vi "stepped_inflation.vi"() -> ()   [LabVIEW 2014]
doc: "This VI demonstrates the individual configuration of settings in I/W, W/I, and continuous operation modes.\n\nThis VI is not meant to be used with infusion-only models. \n\nNotes:\n(1) If continuous mode is selected, infuse volumes/rates will be used."
uses:
  <instrlib>/KD Scientific 2XX Series/KD Scientific 2XX Series.lvlib
panel:
  in  "number of steps":i32
  out "Units":string
  out "Delivered Volume":dbl
  in  "stop":bool
  out "Status":T1
  in  "Baud Rate (9600)":u32(ring)=9600 items=["300"=300, "1200"=1200, "2400"=2400, "4800"=4800, "9600"=9600]
  in  "Withdrawal Settings":T2={"Flow Rate (5)"=5.0, "Volume (10)"=10.0, "Volume Units (ml)"=enum."milliliters (ml)", "Rate Units (ml/min.)"=enum."milliliters per minute (ml/min.)"} {"Volume (10)" format="%#.3g"}
  in  "Diameter (8.75 mm)":dbl=8.75
  in  "Infusion Settings":T2={"Flow Rate (5)"=5.0, "Volume (10)"=10.0, "Volume Units (ml)"=enum."milliliters (ml)", "Rate Units (ml/min.)"=enum."milliliters per minute (ml/min.)"}
  in  "Operation Mode (Infuse)":u16(ring) items=["Infuse", "Withdraw", "Infuse-Withdraw", "Withdraw-Infuse", "Continuous"]
  in  "Address (0)":i32 format="%0.0f"
  in  "error in (no error)":errorcluster
  in  "VISA resource name":refnum<visa-resource-name>="COM1"
  # "© 2005 National Instruments Corporation.  ALL RIGHTS RESERVED."
  # "RS-232 Settings"
  # "General Settings"
  # "Pump Status"
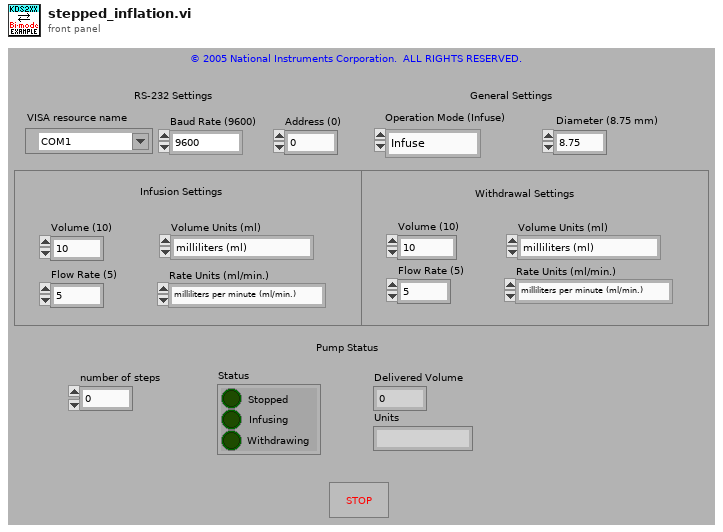
[diagram p1: front panel]
types:
  T1 = cluster{"Stopped":bool, "Infusing":bool, "Withdrawing":bool}
  T2 = cluster{"Flow Rate (5)":dbl, "Volume (10)":dbl, "Volume Units (ml)":enum16{"milliliters (ml)", "microliters (ul)"}, "Rate Units (ml/min.)":enum16{"milliliters per minute (ml/min.)", "milliliters per hour (ml/hr.)", "microliters per minute (ul/min.)", "microliters per hour (ul/hr.)"}}
  T3 = enum16{"milliliters per minute (ml/min.)", "milliliters per hour (ml/hr.)", "microliters per minute (ul/min.)", "microliters per hour (ul/hr.)"}
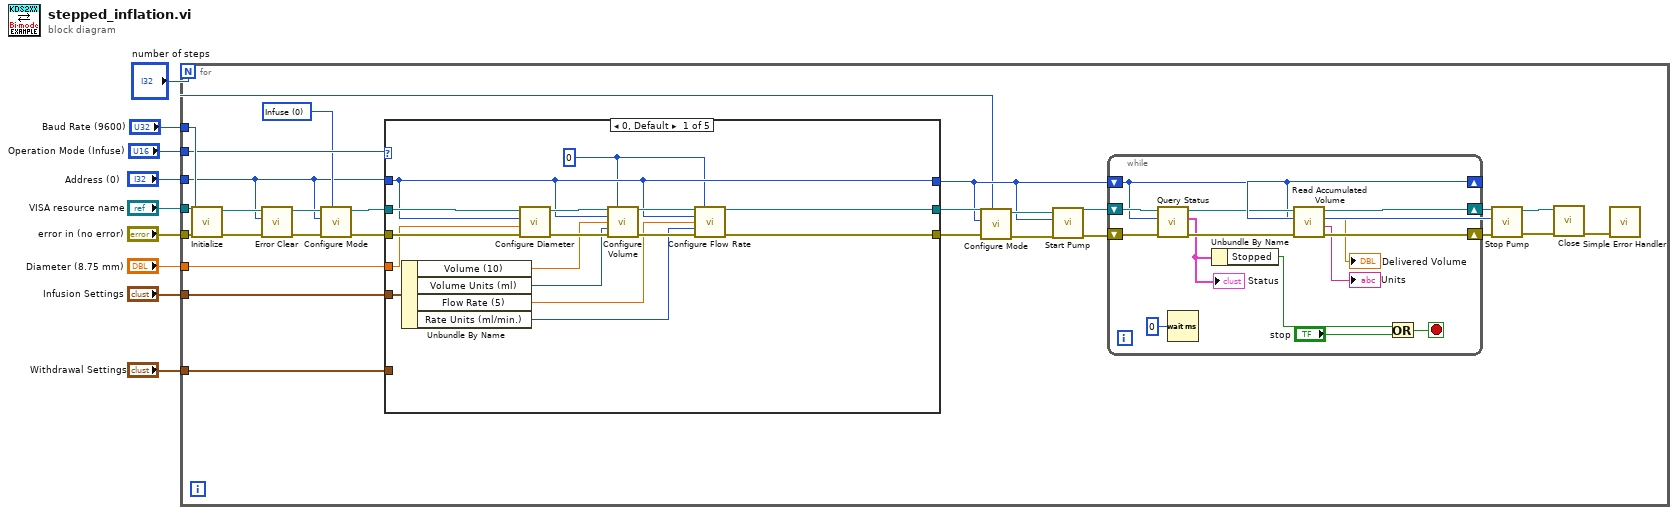
[diagram p0: block diagram]
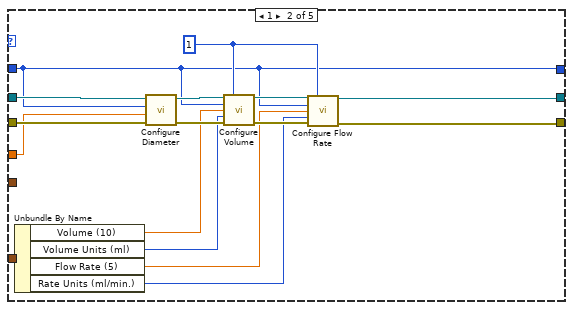
[diagram p2: hidden frame]
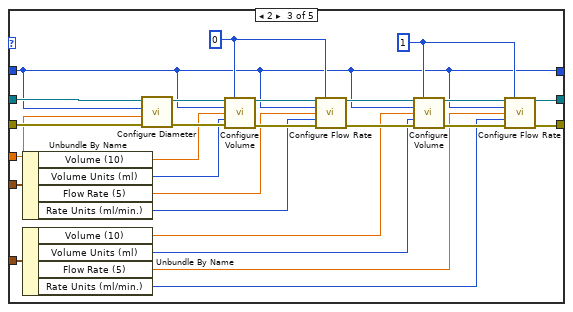
[diagram p3: hidden frame]
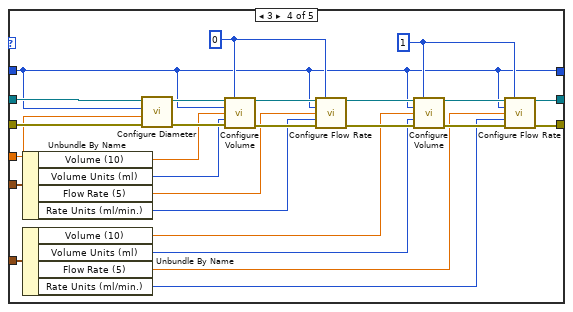
[diagram p4: hidden frame]
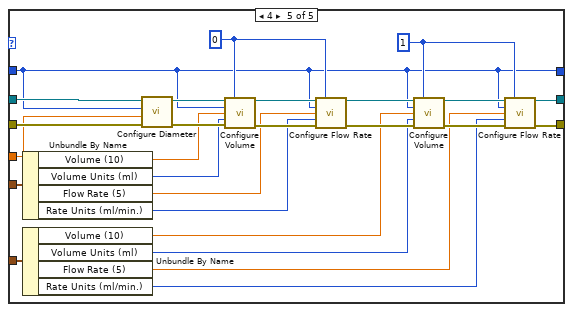
[diagram p5: hidden frame]
diagram:
  n1 = for {
    N: "number of steps" -> [_]
    tunnel: "VISA resource name" -> [w37]
    tunnel: "error in (no error)" -> [w36]
    tunnel: "Infusion Settings" -> [w31]
    tunnel: "Withdrawal Settings" -> [w30]
    tunnel: "Diameter (8.75 mm)" -> [w29]
    tunnel: "Baud Rate (9600)" -> [w24]
    tunnel: "Operation Mode (Infuse)" -> [w18]
    tunnel: "Address (0)" -> [w10]
    w15 = u16 0 items=["Infuse", "Withdraw", "Infuse-Withdraw", "Withdraw-Infuse", "Continuous"] ("Mode (infuse)")
    n2 = call <instrlib>:"Initialize.vi"("error in (no error)"=w36, "Baud Rate (9600)"=w24, "VISA resource name"=w37) -> ("error out"=w12:errorcluster, "VISA resource name out"=w11:refnum<visa-resource-name>)  [unwired: 7 in]
    n3 = call <instrlib>:"Error Clear.vi"("error in (no error)"=w12, "Address (0)"=w10, "VISA resource name"=w11) -> ("error out"=w13:errorcluster, "VISA resource name out"=w14:refnum<visa-resource-name>)  [unwired: 6 in, 1 out]
    n4 = call <instrlib>:"Configure Mode.vi"("Mode (infuse)"=w15, "error in (no error)"=w13, "Address (0)"=w10, "VISA resource name"=w14) -> ("error out"=w17:errorcluster, "VISA resource name out"=w16:refnum<visa-resource-name>)  [unwired: 6 in]
    n5 = case shown="0, Default" w18 {
      tunnel: w31 -> [w47 _ w95 w121 w147]
      tunnel: w30 -> [_ w69 w94 w120 w146]
      tunnel: w16 -> [w53 w68 w93 w119 w145]
      tunnel: w17 -> [w52 w64 w92 w118 w144]
      tunnel: w29 -> [w46 w60 w75 w101 w127]
      tunnel: [w45 w54 w70 w96 w122] -> w19
      tunnel: w10 -> [w45 w54 w70 w96 w122]
      tunnel: [w40 w65 w72 w98 w124] -> w23
      tunnel: [w39 w61 w71 w97 w123] -> w22
      frame 0, Default {
        w38 = 0
        n6 = Unbundle By Name(w47) -> ("Volume (10)"=w44:dbl, "Volume Units (ml)"=w43:enum16{"milliliters (ml)", "microliters (ul)"}, "Flow Rate (5)"=w42:dbl, "Rate Units (ml/min.)"=w41:T3)
        n7 = call <instrlib>:"Configure Diameter.vi"("error in (no error)"=w52, "Diameter (8.75 mm)"=w46, "Address (0)"=w45, "VISA resource name"=w53) -> ("error out"=w50:errorcluster, "VISA resource name out"=w51:refnum<visa-resource-name>)  [unwired: 6 in]
        n8 = call <instrlib>:"Configure Volume.vi"("VISA resource name"=w51, "Mode (infuse)"=w38, "Address (0)"=w45, "Volume (100)"=w44, "Units (0: milliliters)"=w43, "error in (no error)"=w50) -> ("VISA resource name out"=w49:refnum<visa-resource-name>, "error out"=w48:errorcluster)  [unwired: 8 in]
        n9 = call <instrlib>:"Configure Flow Rate.vi"("VISA resource name"=w49, "Mode (infuse)"=w38, "Address (0)"=w45, "Flow Rate (5)"=w42, "Units (0: milliliters per minute)"=w41, "error in (no error)"=w48) -> ("VISA resource name out"=w40:refnum<visa-resource-name>, "error out"=w39:errorcluster)  [unwired: 8 in]
      }
      frame 1 {
        w55 = 1
        n10 = Unbundle By Name(w69) -> ("Volume (10)"=w59:dbl, "Volume Units (ml)"=w58:enum16{"milliliters (ml)", "microliters (ul)"}, "Flow Rate (5)"=w57:dbl, "Rate Units (ml/min.)"=w56:T3)
        n11 = call <instrlib>:"Configure Diameter.vi"("error in (no error)"=w64, "Diameter (8.75 mm)"=w60, "Address (0)"=w54, "VISA resource name"=w68) -> ("error out"=w63:errorcluster, "VISA resource name out"=w67:refnum<visa-resource-name>)  [unwired: 6 in]
        n12 = call <instrlib>:"Configure Volume.vi"("VISA resource name"=w67, "Mode (infuse)"=w55, "Address (0)"=w54, "Volume (100)"=w59, "Units (0: milliliters)"=w58, "error in (no error)"=w63) -> ("VISA resource name out"=w66:refnum<visa-resource-name>, "error out"=w62:errorcluster)  [unwired: 8 in]
        n13 = call <instrlib>:"Configure Flow Rate.vi"("VISA resource name"=w66, "Mode (infuse)"=w55, "Address (0)"=w54, "Flow Rate (5)"=w57, "Units (0: milliliters per minute)"=w56, "error in (no error)"=w62) -> ("VISA resource name out"=w65:refnum<visa-resource-name>, "error out"=w61:errorcluster)  [unwired: 8 in]
      }
      frame 2 {
        w73 = 1
        w74 = 0
        n14 = Unbundle By Name(w95) -> ("Volume (10)"=w83:dbl, "Volume Units (ml)"=w82:enum16{"milliliters (ml)", "microliters (ul)"}, "Flow Rate (5)"=w81:dbl, "Rate Units (ml/min.)"=w80:T3)
        n15 = Unbundle By Name(w94) -> ("Volume (10)"=w79:dbl, "Volume Units (ml)"=w78:enum16{"milliliters (ml)", "microliters (ul)"}, "Flow Rate (5)"=w77:dbl, "Rate Units (ml/min.)"=w76:T3)
        n16 = call <instrlib>:"Configure Diameter.vi"("error in (no error)"=w92, "Diameter (8.75 mm)"=w75, "Address (0)"=w70, "VISA resource name"=w93) -> ("error out"=w87:errorcluster, "VISA resource name out"=w91:refnum<visa-resource-name>)  [unwired: 6 in]
        n17 = call <instrlib>:"Configure Volume.vi"("VISA resource name"=w91, "Mode (infuse)"=w74, "Address (0)"=w70, "Volume (100)"=w83, "Units (0: milliliters)"=w82, "error in (no error)"=w87) -> ("VISA resource name out"=w90:refnum<visa-resource-name>, "error out"=w86:errorcluster)  [unwired: 8 in]
        n18 = call <instrlib>:"Configure Flow Rate.vi"("VISA resource name"=w90, "Mode (infuse)"=w74, "Address (0)"=w70, "Flow Rate (5)"=w81, "Units (0: milliliters per minute)"=w80, "error in (no error)"=w86) -> ("VISA resource name out"=w89:refnum<visa-resource-name>, "error out"=w85:errorcluster)  [unwired: 8 in]
        n19 = call <instrlib>:"Configure Volume.vi"("VISA resource name"=w89, "Mode (infuse)"=w73, "Address (0)"=w70, "Volume (100)"=w79, "Units (0: milliliters)"=w78, "error in (no error)"=w85) -> ("VISA resource name out"=w88:refnum<visa-resource-name>, "error out"=w84:errorcluster)  [unwired: 8 in]
        n20 = call <instrlib>:"Configure Flow Rate.vi"("VISA resource name"=w88, "Mode (infuse)"=w73, "Address (0)"=w70, "Flow Rate (5)"=w77, "Units (0: milliliters per minute)"=w76, "error in (no error)"=w84) -> ("VISA resource name out"=w72:refnum<visa-resource-name>, "error out"=w71:errorcluster)  [unwired: 8 in]
      }
      frame 3 {
        w99 = 1
        w100 = 0
        n21 = Unbundle By Name(w121) -> ("Volume (10)"=w109:dbl, "Volume Units (ml)"=w108:enum16{"milliliters (ml)", "microliters (ul)"}, "Flow Rate (5)"=w107:dbl, "Rate Units (ml/min.)"=w106:T3)
        n22 = Unbundle By Name(w120) -> ("Volume (10)"=w105:dbl, "Volume Units (ml)"=w104:enum16{"milliliters (ml)", "microliters (ul)"}, "Flow Rate (5)"=w103:dbl, "Rate Units (ml/min.)"=w102:T3)
        n23 = call <instrlib>:"Configure Diameter.vi"("error in (no error)"=w118, "Diameter (8.75 mm)"=w101, "Address (0)"=w96, "VISA resource name"=w119) -> ("error out"=w113:errorcluster, "VISA resource name out"=w117:refnum<visa-resource-name>)  [unwired: 6 in]
        n24 = call <instrlib>:"Configure Volume.vi"("VISA resource name"=w117, "Mode (infuse)"=w100, "Address (0)"=w96, "Volume (100)"=w109, "Units (0: milliliters)"=w108, "error in (no error)"=w113) -> ("VISA resource name out"=w116:refnum<visa-resource-name>, "error out"=w112:errorcluster)  [unwired: 8 in]
        n25 = call <instrlib>:"Configure Flow Rate.vi"("VISA resource name"=w116, "Mode (infuse)"=w100, "Address (0)"=w96, "Flow Rate (5)"=w107, "Units (0: milliliters per minute)"=w106, "error in (no error)"=w112) -> ("VISA resource name out"=w115:refnum<visa-resource-name>, "error out"=w111:errorcluster)  [unwired: 8 in]
        n26 = call <instrlib>:"Configure Volume.vi"("VISA resource name"=w115, "Mode (infuse)"=w99, "Address (0)"=w96, "Volume (100)"=w105, "Units (0: milliliters)"=w104, "error in (no error)"=w111) -> ("VISA resource name out"=w114:refnum<visa-resource-name>, "error out"=w110:errorcluster)  [unwired: 8 in]
        n27 = call <instrlib>:"Configure Flow Rate.vi"("VISA resource name"=w114, "Mode (infuse)"=w99, "Address (0)"=w96, "Flow Rate (5)"=w103, "Units (0: milliliters per minute)"=w102, "error in (no error)"=w110) -> ("VISA resource name out"=w98:refnum<visa-resource-name>, "error out"=w97:errorcluster)  [unwired: 8 in]
      }
      frame 4 {
        w125 = 1
        w126 = 0
        n28 = Unbundle By Name(w147) -> ("Volume (10)"=w135:dbl, "Volume Units (ml)"=w134:enum16{"milliliters (ml)", "microliters (ul)"}, "Flow Rate (5)"=w133:dbl, "Rate Units (ml/min.)"=w132:T3)
        n29 = Unbundle By Name(w146) -> ("Volume (10)"=w131:dbl, "Volume Units (ml)"=w130:enum16{"milliliters (ml)", "microliters (ul)"}, "Flow Rate (5)"=w129:dbl, "Rate Units (ml/min.)"=w128:T3)
        n30 = call <instrlib>:"Configure Diameter.vi"("error in (no error)"=w144, "Diameter (8.75 mm)"=w127, "Address (0)"=w122, "VISA resource name"=w145) -> ("error out"=w139:errorcluster, "VISA resource name out"=w143:refnum<visa-resource-name>)  [unwired: 6 in]
        n31 = call <instrlib>:"Configure Volume.vi"("VISA resource name"=w143, "Mode (infuse)"=w126, "Address (0)"=w122, "Volume (100)"=w135, "Units (0: milliliters)"=w134, "error in (no error)"=w139) -> ("VISA resource name out"=w142:refnum<visa-resource-name>, "error out"=w138:errorcluster)  [unwired: 8 in]
        n32 = call <instrlib>:"Configure Flow Rate.vi"("VISA resource name"=w142, "Mode (infuse)"=w126, "Address (0)"=w122, "Flow Rate (5)"=w133, "Units (0: milliliters per minute)"=w132, "error in (no error)"=w138) -> ("VISA resource name out"=w141:refnum<visa-resource-name>, "error out"=w137:errorcluster)  [unwired: 8 in]
        n33 = call <instrlib>:"Configure Volume.vi"("VISA resource name"=w141, "Mode (infuse)"=w125, "Address (0)"=w122, "Volume (100)"=w131, "Units (0: milliliters)"=w130, "error in (no error)"=w137) -> ("VISA resource name out"=w140:refnum<visa-resource-name>, "error out"=w136:errorcluster)  [unwired: 8 in]
        n34 = call <instrlib>:"Configure Flow Rate.vi"("VISA resource name"=w140, "Mode (infuse)"=w125, "Address (0)"=w122, "Flow Rate (5)"=w129, "Units (0: milliliters per minute)"=w128, "error in (no error)"=w136) -> ("VISA resource name out"=w124:refnum<visa-resource-name>, "error out"=w123:errorcluster)  [unwired: 8 in]
      }
    }
    n35 = call <instrlib>:"Configure Mode.vi"("Mode (infuse)"=w18, "error in (no error)"=w22, "Address (0)"=w19, "VISA resource name"=w23) -> ("error out"=w20:errorcluster, "VISA resource name out"=w21:refnum<visa-resource-name>)  [unwired: 6 in]
    n36 = call <instrlib>:"Start Pump.vi"("error in (no error)"=w20, "Address (0)"=w19, "VISA resource name"=w21) -> ("error out"=w34:errorcluster, "VISA resource name out"=w35:refnum<visa-resource-name>)  [unwired: 7 in]
    n37 = while {
      shift-right: [w150] -> w28
      shift-left: w19 -> [w150]
      shift-right: [w152] -> w33
      shift-left: w35 -> [w158]
      shift-right: [w151] -> w32
      shift-left: w34 -> [w159]
      stop <- w156 stop-if-true
      n38 = call <instrlib>:"Query Status.vi"("error in (no error)"=w159, "Address (0)"=w150, "VISA resource name"=w158) -> ("error out"=w161:errorcluster, "Status"=w157:T1, "VISA resource name out"=w153:refnum<visa-resource-name>)  [unwired: 6 in]
      "Status" <- w157
      n39 = Wait (ms)(milliseconds to wait=u32 0) -> ()  [unwired: 1 out]
      n40 = Unbundle By Name(w157) -> ("Stopped"=w155:bool)
      n41 = call <instrlib>:"Read Accumulated Volume.vi"("error in (no error)"=w161, "Address (0)"=w150, "VISA resource name"=w153) -> ("error out"=w151:errorcluster, "Units"=→"Units":string, "Delivered Volume"=→"Delivered Volume":dbl, "VISA resource name out"=w152:refnum<visa-resource-name>)  [unwired: 5 in]
      n42 = Or(x=w155, y="stop") -> (x .or. y?=w156:bool)
    }
    n43 = call <instrlib>:"Stop Pump.vi"("error in (no error)"=w32, "Address (0)"=w28, "VISA resource name"=w33) -> ("error out"=w26:errorcluster, "VISA resource name out"=w25:refnum<visa-resource-name>)  [unwired: 7 in]
    n44 = call <instrlib>:"Close.vi"("error in (no error)"=w26, "VISA resource name"=w25) -> ("error out"=w27:errorcluster)  [unwired: 9 in]
    n45 = call <vilib>:"Simple Error Handler.vi"("error in (no error)"=w27) -> ()  [unwired: 4 in, 5 out]
  }
